vi "SR1.start scan.vi"(0 "i ref in":refnum<vi>, 5 "error in (no error)":errorcluster) -> (14 "i ref out":refnum<vi>, 19 "error out":errorcluster)   [LabVIEW 2014, in "SR1.lvlib"]
doc: "starts a scan (or: starts waiting for a trigger to start)"
uses:
  SR1.lvlib
  CS_Core/CSSystem/CoreDefs/CoreDefs.error_type.ctl
  CS_Core/CSSystem/CoreLib/CoreLib.lvlib
  CSlibraries/UtilityLib/UtilityLib.lvlib
  instr.lib/Stanford Research SR1/Stanford Research SR1.lvlib
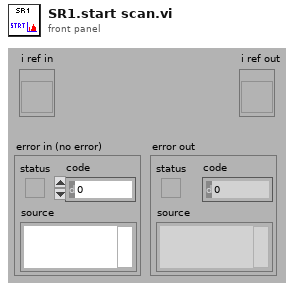
[diagram p1: front panel]
types:
  T1 = typedef "CoreDefs.error_type.ctl" = enum16{"no error", "can't load process", "can't unload process", "process does not exist", "can't install process", "can't remove process", "unknown function", "time out", "can't execute function", "duplicate queue name", "super not found", "caller queue invalid", "can't ping process", "unknown error", "VISA Error", "VISA timeout", "GPIB timeout", "GPIB error", "communication error", "data type mismatch", "can't read data from OPC server", "can't write data to OPC server", "OET error", "function not implemented", "process already exists", "invalid Shared Variable name", "error writing Shared Variable", "error reading Shared Variable", "invalid client name", "corrupt database", "unknown class", "call not authorized", "parameter out of range", "OET timeout: can't get data to modify", "invalid queue name", "requested operation incompatible with current state", "event undefined", "event disabled", "state undefined", "caller is not a friend", "EventBuilder: bad eventID", "EventBuilder: no DAQ devices", "a thread must not stop itself", "UNUSED ELEMENT4", "DiscArchiver: eventData incomplete", "DiscArchiver: eventData does not belong to run", "DiscArchiver: can't open file", "DiscArchiver: can't write to file", "DiscArchiver: available disc space low", "can't acquire semaphore", "error reading data from database", "notifier object is not existing", "can't register process", "can't unregister process", "illegal event type", "object disabled", "object already exists", "can't change state", "Instrument not found", "no connection to remote node", "invalid reference", "N/A", "UNUSED ELEMENT 1", "element not found", "illegal TCP/IP connection detected", "object does not exist", "invalid access ID", "unknown CS system", "invalid privilige", "unsupported data type", "unsupported server type", "IO server already exists", "Shared Variable already exists"}
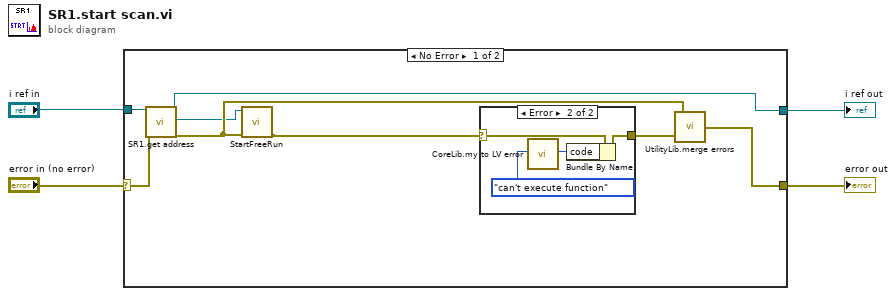
[diagram p0: block diagram]
diagram:
  n1 = case shown="No Error" "error in (no error)" {
    selector: "error in (no error)" -> [w7 w18]
    tunnel: "i ref in" -> [w12 w19]
    tunnel: [w10 w18] -> w3
    tunnel: [w9 w19] -> w2
    frame No Error {
      n2 = call "SR1.get address.vi"("i ref in"=w12, "error in (no error)"=w7) -> ("i ref out"=w9:refnum<vi>, "VISA resource name"=w6:refnum<visa-resource-name>, "error out"=w11:errorcluster)  [unwired: 15 in]
      n3 = call "StartFreeRun.vi"("error in (no error)"=w11, "VISA resource name"=w6) -> ("error out"=w5:errorcluster)  [unwired: 8 in, 1 out]
      n4 = case shown="Error" w5 {
        selector: w5 -> [w13 w17]
        tunnel: [w13 w14] -> w8
        frame No Error {
        }
        frame Error {
          n5 = call "CoreLib.my to LV error.vi"("ErrorTypes"=CoreDefs.error_type."can't execute function") -> ("LV error code"=w16:i32)  [unwired: 17 in, 1 out]
          n6 = Bundle By Name(cluster=w17, "code"=w16) -> (w14:errorcluster)
        }
      }
      n7 = call "UtilityLib.merge errors.vi"("error2 (no error)"=w8, "error1 (no error)"=w11) -> ("error out"=w10:errorcluster)
    }
    frame Error {
    }
  }
  "error out" <- w3
  "i ref out" <- w2
